vi "Construct Model Synchronously Requests Double Float.vi"(9 "DBL Request Timeout (2000)":i32=2000, 11 "DBL Name":string) -> (1 "Result Notifier":refnum<notifier>, 3 "ModelSynchronouslyRequestsDoubleFloat Out":refnum<class "ModelSynchronouslyRequestsDoubleFloat.lvclass">)   [LabVIEW 2017, in "ModelSynchronouslyRequestsDoubleFloat.lvclass"]
uses:
  ModelSynchronouslyRequestsDoubleFloat.lvclass
  ModelSynchronouslyRequestsDoubleFloat.lvclass/ModelSynchronouslyRequestsDoubleFloat.ctl
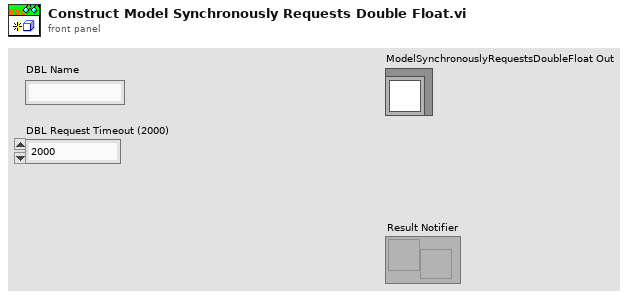
[diagram p1: front panel]
types:
  T1 = cluster{"Received Value":dbl, "Timed Out?":bool, "Sync Request Error":errorcluster}
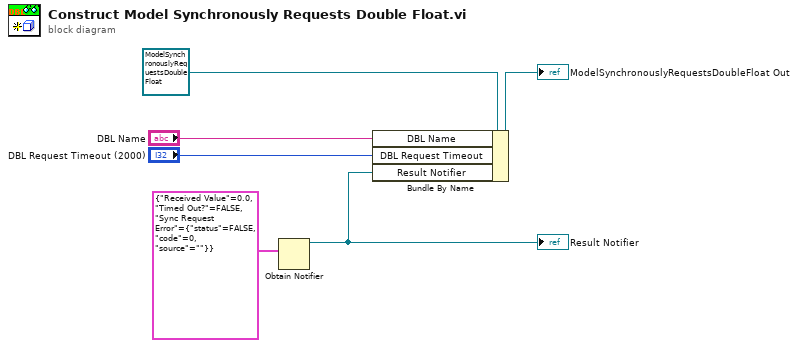
[diagram p0: block diagram]
diagram:
  n1 = Obtain Notifier(notification data type=T1 {"Received Value"=0.0, "Timed Out?"=FALSE, "Sync Request Error"={"status"=FALSE, "code"=0, "source"=""}}) -> (notifier out=w2:refnum<notifier>)  [unwired: 3 in, 2 out]
  "Result Notifier" <- w2
  n2 = Bundle By Name(cluster=refnum<class "ModelSynchronouslyRequestsDoubleFloat.lvclass"> refnum ("ModelLeaksStateAfterLaunch in"), "DBL Name"="DBL Name", "DBL Request Timeout"="DBL Request Timeout (2000)", "Result Notifier"=w2) -> (→"ModelSynchronouslyRequestsDoubleFloat Out":refnum<class "ModelSynchronouslyRequestsDoubleFloat.lvclass">)
